vi "GoHome.vi"(8 "error in (no error)":errorcluster, 10 "Axis":enum16{"X", "Y", "Z", "HOM"}(ring), 11 "TranslationStageUI.lvclass":refnum<class "TranslationStageUI.lvclass">) -> (0 "error out":errorcluster, 3 "TranslationStageUI.lvclass":refnum<class "TranslationStageUI.lvclass">)   [LabVIEW 2023, in "TranslationStageUI.lvclass"]
uses:
  TranslationStageUI.lvclass
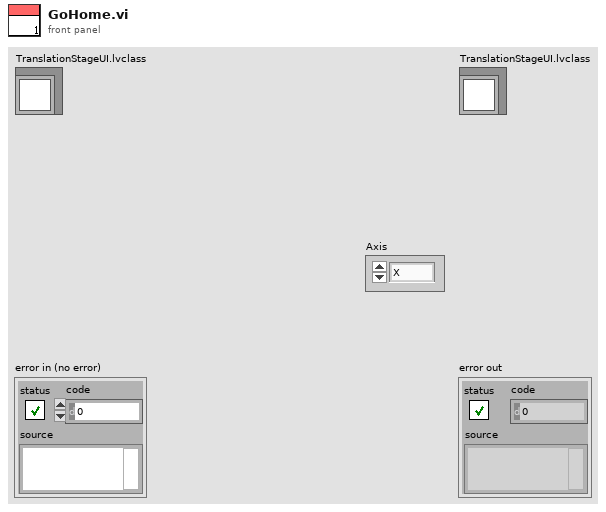
[diagram p1: front panel]
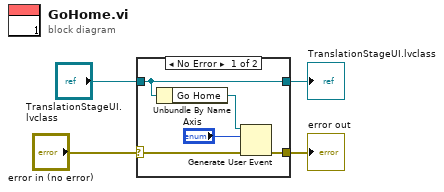
[diagram p0: block diagram]
diagram:
  n1 = case shown="No Error" "error in (no error)" {
    selector: "error in (no error)" -> [w6 w11]
    tunnel: [w5 w11] -> w3
    tunnel: [w9 w10] -> w1
    tunnel: "TranslationStageUI.lvclass" -> [w9 w10]
    frame No Error {
      n2 = Unbundle By Name(w9) -> ("Go Home"=w8:refnum<user-event>)
      n3 = Generate User Event(user event=w8, event data cluster="Axis", error in=w6) -> (error out=w5:errorcluster)  [unwired: 1 in, 1 out]
    }
    frame Error {
    }
  }
  "error out" <- w3
  "TranslationStageUI.lvclass" <- w1
